vi "AutoElevReadyWait.vi"(8 "error in (no error)":errorcluster, 10 "ElevatorSetpoints":T1=enum."Rest", 11 "TimeOut (s)":dbl=99.0) -> (0 "error out":errorcluster)   [LabVIEW 2023]
doc: "Wrapper class for auto do nothing and wait\nInput:\n -- error in -- Cluster \n -- time out -- Double -- how long to wait B4 quitting\nOutput:\n -- error out -- Cluster"
uses:
  Elevator/ElevatorSetpointEnum.ctl
  <vilib>/Rock Robotics/WPI/ThirdParty/JAS_Junk/TrajLib/ChassisSpeeds_New.vi
  <vilib>/Rock Robotics/WPI/ThirdParty/JAS_Junk/TrajLib/Conv_Feet_Meters.vi
  <vilib>/Rock Robotics/WPI/ThirdParty/JAS_Junk/TrajLib/Conv_Deg_Radians.vi
  Elevator/ElevatorSetpoints.vi
  Elevator/ElevatorGetPosition.vi
  Wrist/WristAtSetpoint.vi
  <vilib>/Utility/semaphor.llb/Obtain Semaphore Reference.vi
  <vilib>/Rock Robotics/WPI/ThirdParty/JAS_Junk/TrajLib/Timer_Reset.vi
  Drive/DriveGlobal.vi
  Wrist/WristGlobal.vi
  Elevator/ElevatorGlobal.vi
  <vilib>/Rock Robotics/WPI/ThirdParty/JAS_Junk/TrajLib/Trajectory_Library.lvlib
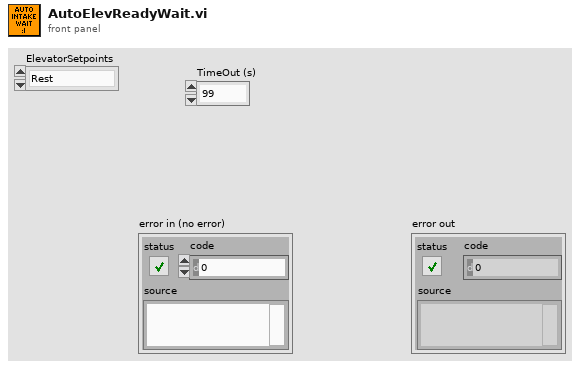
[diagram p1: front panel]
types:
  T1 = typedef "ElevatorSetpointEnum.ctl" = enum16{"Floor", "Rest", "Source", "L1", "L2", "Algae1", "L3", "Algae2", "L4", "Barge", "Processor"}
  T2 = typedef "Trajectory_Library.lvlib/TIMER.ctl" = cluster{"StartTime":dbl, "Accumulated TIme":dbl, "Running":bool, "semaphore":T3}
  T3 = typedef "Semaphore RefNum" = refnum<k1>
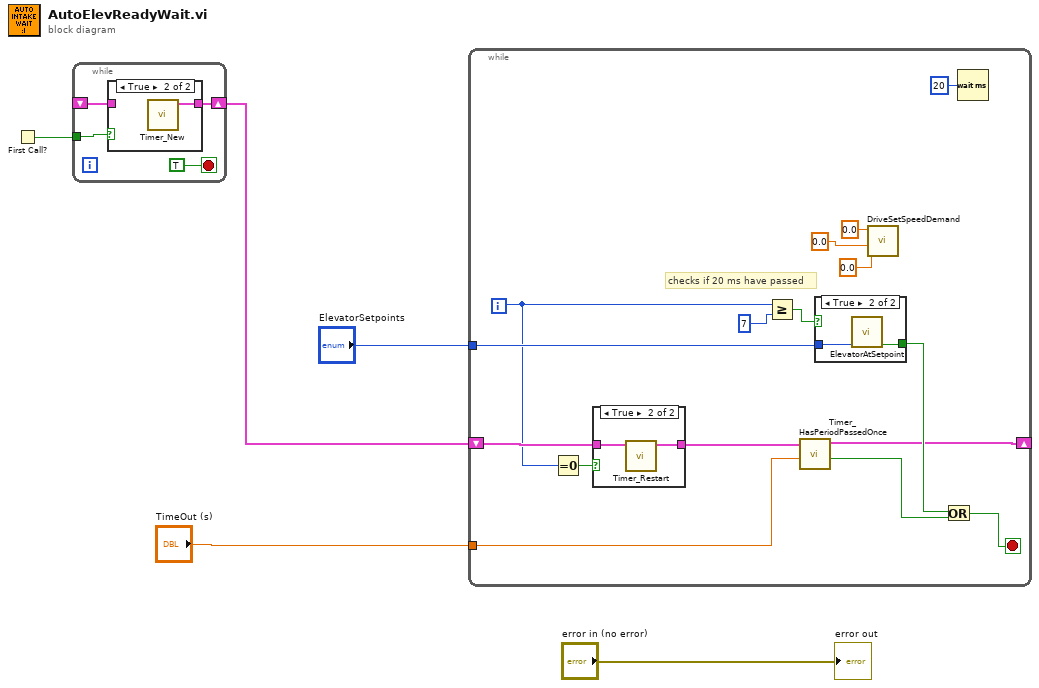
[diagram p0: block diagram]
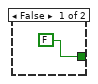
[diagram p4: hidden frame]
diagram:
  n1 = First Call?() -> (First Call?: T/F=w2:bool)
  n2 = while {
    tunnel: w2 -> [w6]
    shift-right: [w9] -> w1
    shift-left: _ -> [w7]
    stop <- TRUE stop-if-true
    n3 = case shown="True" w6 {
      tunnel: [w10 w11] -> w9
      tunnel: w7 -> [w10 _]
      frame False {
      }
      frame True {
        n4 = call <vilib>:"Timer_New.vi"() -> ("TIMER"=w11:T2)  [unwired: 11 in]
      }
    }
  }
  n5 = while {
    tunnel: "TimeOut (s)" -> [w27]
    tunnel: "ElevatorSetpoints" -> [w17]
    shift-right: [w16] -> _
    shift-left: w1 -> [w13]
    i -> [w12]
    stop <- w20 stop-if-true
    # "checks if 20 ms have passed"
    n6 = Equal To 0?(x=w12) -> (x = 0?=w15:bool)
    n7 = case shown="True" w15 {
      tunnel: w13 -> [w28 w30]
      tunnel: [w28 w29] -> w14
      frame False {
      }
      frame True {
        n8 = call <vilib>:"Timer_Restart.vi"("in Timer"=w30) -> ("out Timer"=w29:T2)  [unwired: 10 in]
      }
    }
    n9 = Greater Or Equal?(x=w12, y=7) -> (x >= y?=w19:bool)
    n10 = call <vilib>:"Timer_HasPeriodPassedOnce.vi"("Period"=w27, "in Timer"=w14) -> ("Expired"=w21:bool, "out Timer"=w16:T2)  [unwired: 7 in, 1 out]
    n11 = case shown="True" w19 {
      tunnel: [FALSE w33] -> w22
      tunnel: w17 -> [_ w32]
      frame False {
      }
      frame True {
        n12 = call "ElevatorAtSetpoint.vi"("ElevatorSetpoints"=w32) -> ("AtSetpoint"=w33:bool)  [unwired: 10 in]
      }
    }
    n13 = call "DriveSetSpeedDemand.vi"("ASpeedDemand (d/s)"=0.0 ("RSpeedDemand (ft/s)"), "YSpeedDemand (ft/s)"=0.0 ("RSpeedDemand (ft/s)"), "XSpeedDemand (ft/s)"=0.0 ("LSpeedDemand (ft/s)")) -> ()  [unwired: 9 in]
    n14 = Or(x=w22, y=w21) -> (x .or. y?=w20:bool)
    n15 = Wait (ms)(milliseconds to wait=u32 20) -> ()  [unwired: 1 out]
  }
  "error out" <- "error in (no error)"
